vi "Add Found Resolver to Aarray.vi"(7 "Index Found":i32, 8 "Controls In":T1[](array[typedef]), 9 "ScaleFactor 1 Name":string, 10 "Resolver Number":string, 11 "Resolvers In":T2[](array[typedef])) -> (2 "Controls Out":T1[](array[typedef]), 3 "Resolvers Out":T2[](array[typedef]), 5 "Next Index":i32)   [LabVIEW 2011, in "Sensor Simulation Custom Device.lvlib"]
uses:
  Sensor Simulation Custom Device.lvlib
  <userlib>/_FPGA Interface Advanced Tools/FPGA Bitfile Utility/TypeDefs/Scalar Register.ctl
  TypeDefs/Resolver.ctl
  <userlib>/_FPGA Interface Advanced Tools/FPGA Bitfile Utility/FPGA Bitfile Utility.lvlib
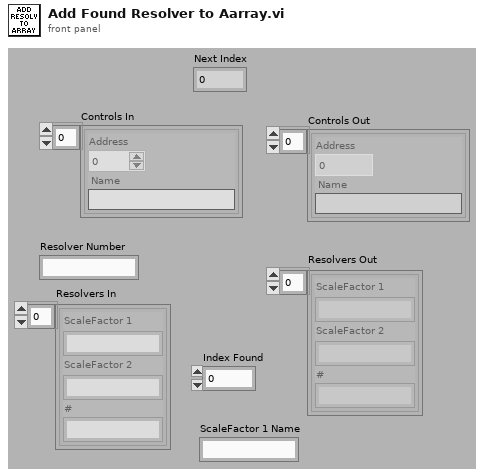
[diagram p1: front panel]
types:
  T1 = typedef "FPGA Bitfile Utility.lvlib/Scalar Register.ctl" = cluster{"Address":u32, "Name":string}
  T2 = typedef "Sensor Simulation Custom Device.lvlib/Resolver.ctl" = cluster{"ScaleFactor 1":string, "ScaleFactor 2":string, "#":string}
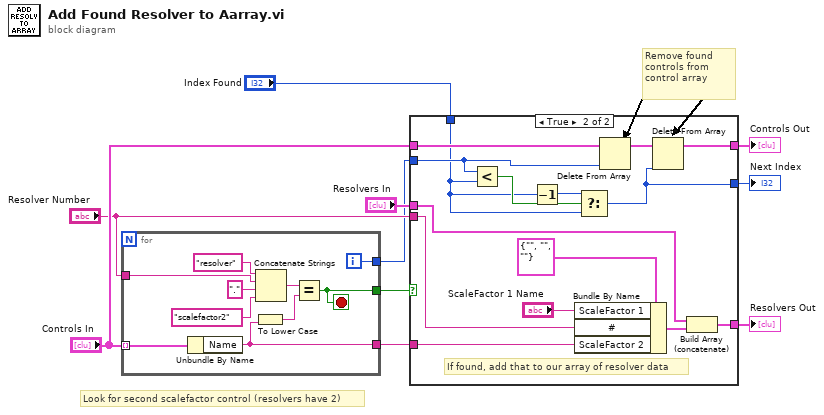
[diagram p0: block diagram]
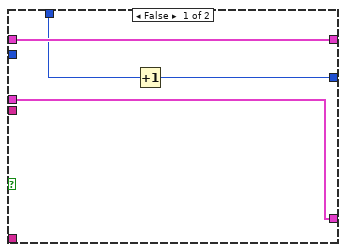
[diagram p2: hidden frame]
diagram:
  # "Remove found controls from control array"
  # "Look for second scalefactor control (resolvers have 2)"
  n1 = for {
    tunnel: [w14] -> w10
    tunnel: [w16] -> w9
    tunnel: [w15] -> w2
    tunnel: "Controls In" -> [w11] mode=indexing
    tunnel: "Resolver Number" -> [w13]
    i -> [w15]
    stop <- w14 stop-if-true
    n2 = Unbundle By Name(w11) -> ("Name"=w16:string)
    n3 = To Lower Case(string=w16) -> (all lower case string=w20:string)
    n4 = Concatenate Strings("resolver" ("regular expression"), w13, "." ("string"), "scalefactor2" ("regular expression")) -> (w17:string)
    n5 = Equal?(x=w17, y=w20) -> (x = y?=w14:bool)
  }
  n6 = case shown="True" w10 {
    tunnel: w9 -> [_ w39]
    tunnel: "Controls In" -> [w24 w38]
    tunnel: w2 -> [_ w29]
    tunnel: [w24 w33] -> w8
    tunnel: "Resolver Number" -> [_ w35]
    tunnel: "Resolvers In" -> [w23 w32]
    tunnel: [w23 w30] -> w4
    tunnel: "Index Found" -> [w22 w26]
    tunnel: [w21 w25] -> w1
    frame False {
      n7 = Increment(x=w22) -> (x+1=w21:i32)
    }
    frame True {
      # "If found, add that to our array of resolver data"
      n8 = Less?(x=w29, y=w26) -> (x < y?=w28:bool)
      n9 = Decrement(x=w26) -> (x-1=w27:i32)
      n10 = Bundle By Name(cluster=T2 {"ScaleFactor 1"="", "ScaleFactor 2"="", "#"=""}, "ScaleFactor 1"="ScaleFactor 1 Name", "#"=w35, "ScaleFactor 2"=w39) -> (w31:T2)
      n11 = Select(t=w27, s=w28, f=w26) -> (s? t:f=w25:i32)
      n12 = Delete From Array(array=w38, index=w29) -> (array with subset deleted=w34:T1[])  [unwired: 1 in, 1 out]
      n13 = Delete From Array(array=w34, index=w25) -> (array with subset deleted=w33:T1[])  [unwired: 1 in, 1 out]
      n14 = Build Array (concatenate)(w32, w31) -> (w30:T2[])
    }
  }
  "Resolvers Out" <- w4
  "Controls Out" <- w8
  "Next Index" <- w1
